vi "Get Blob Snapshot Metadata.vi"(7 "Snapshot":string, 8 "error in (no error)":errorcluster, 9 "Blob":string, 10 "Container":string, 11 "Azure Session in":refnum<class "Session.lvclass">) -> (0 "error out":errorcluster, 2 "Blob Metadata":T1[](array[typedef]), 3 "Azure Session out":refnum<class "Session.lvclass">)   [LabVIEW 2015, in "NI_Azure_Blob.lvlib"]
doc: "Retrieves all user-defined metadata of an existing snapshot of a blob."
uses:
  NI_Azure_Blob.lvlib
  Core/Session/Session.lvclass
  Core/Name Value Pair.ctl
  Core/Session/Session.lvclass/Session.ctl
  Core/Session/Write HTTP Verb.vi
  Core/Session/Write URL Suffix.vi
  Core/Session/Write Request Parameters.vi
  Core/NI_Azure_Core.lvlib
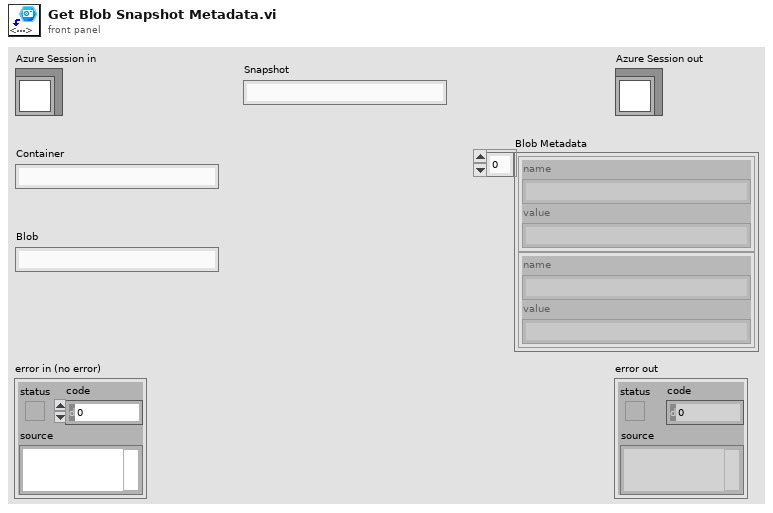
[diagram p1: front panel]
types:
  T1 = typedef "NI_Azure_Core.lvlib/Name Value Pair.ctl" = cluster{"name":string, "value":string}
  T2 = typedef "NI_Azure_Core.lvlib/Response.ctl" = cluster{"Headers":string, "Body":string}
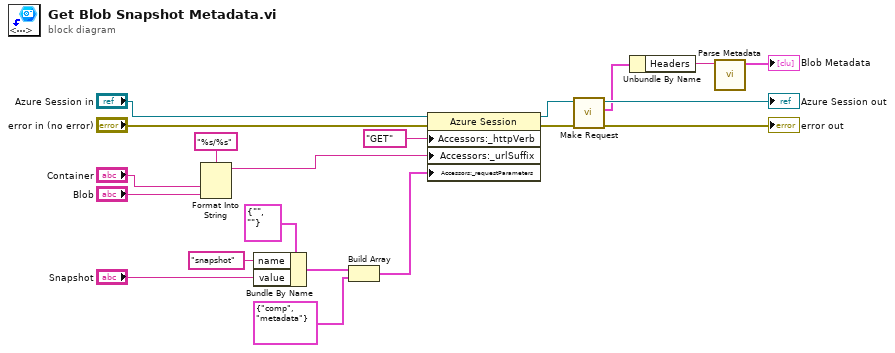
[diagram p0: block diagram]
diagram:
  n1 = Format Into String(format string="%s/%s", "Container", "Blob") -> (resulting string=w7:string)  [unwired: 2 in, 1 out]
  n2 = Bundle By Name(cluster=T1 {"name"="", "value"=""} ("Name Value Pair"), "name"="snapshot", "value"="Snapshot") -> (w4:T1)
  n3 = Build Array(w4, T1 {"name"="comp", "value"="metadata"} ("Name Value Pair")) -> (w1:T1[])
  n4 = property class="Azure Session"(reference="Azure Session in", error in="error in (no error)", "Accessors:_httpVerb"="GET" ("HTTP-Verb"), "Accessors:_urlSuffix"=w7, "Accessors:_requestParameters"=w1) -> (reference out=w9:refnum<class "Session.lvclass">, error out=w11:errorcluster)
  n5 = call "Make Request.vi"("error in (no error)"=w11, "Session in"=w9) -> ("error out"=→"error out":errorcluster, "Response"=w12:T2, "Session out"=→"Azure Session out":refnum<class "Session.lvclass">)  [unwired: 7 in]
  n6 = Unbundle By Name(w12) -> ("Headers"=w13:string)
  n7 = call "Parse Metadata.vi"("String"=w13) -> ("Metadata"=→"Blob Metadata":T1[])  [unwired: 10 in]
